vi "Write Running Actors.vi"(6 "Debug Ring Value":u16, 8 "error in (no error)":errorcluster, 10 "Running Actors":refnum<class "CO2 Actor.lvclass">[](array[class]), 11 "cRIO-CO2 in":refnum<class "cRIO-CO2.lvclass">) -> (0 "error out":errorcluster, 3 "cRIO-CO2 out":refnum<class "cRIO-CO2.lvclass">)   [LabVIEW 2015, in "cRIO-Carbondioxide.lvlib" / "cRIO-CO2.lvlib" / "cRIO-CO2.lvclass"]
uses:
  cRIO-CO2.lvclass
  CO2 Actor/CO2 Actor.lvclass
  CO2 Actor/CO2 Actor.lvclass/CO2 Actor.ctl
  <vilib>/ActorFramework/Actor/Actor.lvclass/Actor.ctl
  <vilib>/ActorFramework/Message Enqueuer/Message Enqueuer.lvclass/Message Enqueuer.ctl
  CO2 Actor Messages/Set IndexQ Msg/Set IndexQ Msg.lvclass/Set IndexQ Msg.ctl
  cRIO-CO2.lvclass/cRIO-CO2.ctl
  <vilib>/ActorFramework/Actor/Read Self Enqueuer.vi
  <vilib>/ActorFramework/Message Enqueuer/Enqueue.vi
  <vilib>/ActorFramework/Message Enqueuer/Init from Existing Queue.vi
  <vilib>/ActorFramework/Message Priority Queue/Priority Enqueue.vi
  <vilib>/ActorFramework/Actor/Actor.lvclass
  <vilib>/ActorFramework/Message Enqueuer/Message Enqueuer.lvclass
  CO2 Actor Messages/Set IndexQ Msg/Set IndexQ Msg.lvclass
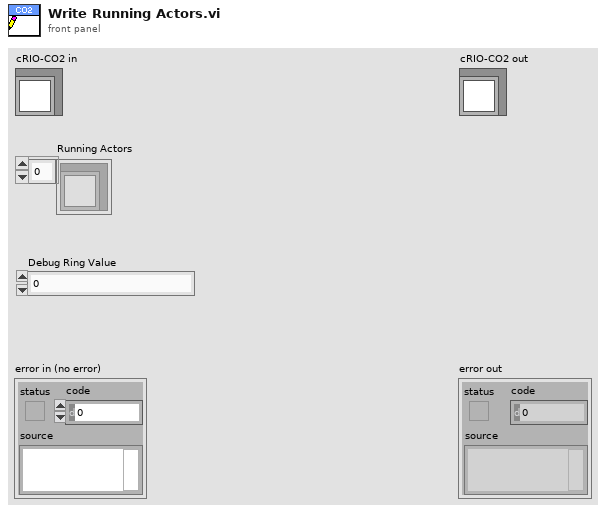
[diagram p1: front panel]
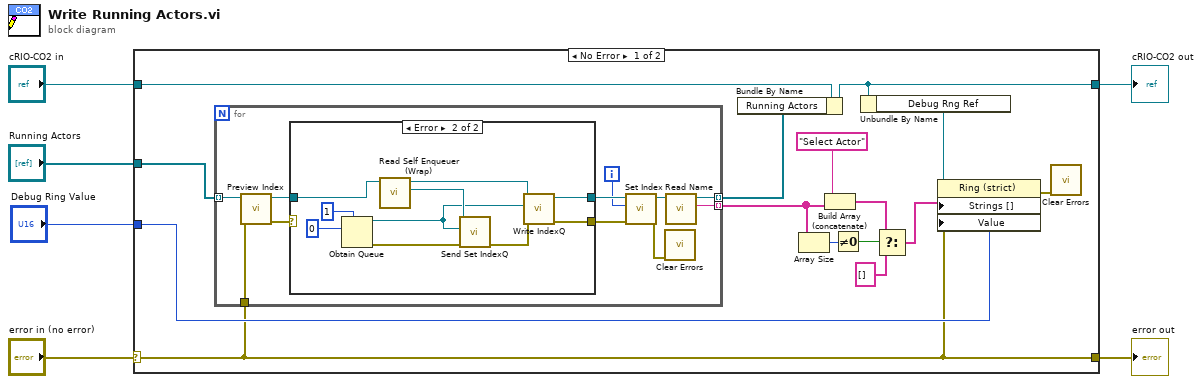
[diagram p0: block diagram]
diagram:
  n1 = case shown="No Error" "error in (no error)" {
    selector: "error in (no error)" -> [w10 w45]
    tunnel: [w10 w45] -> w5
    tunnel: [w8 w46] -> w3
    tunnel: "cRIO-CO2 in" -> [w9 w46]
    tunnel: "Running Actors" -> [w21 _]
    tunnel: "Debug Ring Value" -> [w17 _]
    frame No Error {
      n2 = for {
        tunnel: w21 -> [w29] mode=indexing
        tunnel: [w32] -> w16 mode=indexing
        tunnel: w10 -> [w28]
        tunnel: [w22] -> w7 mode=indexing
        i -> [w23]
        n3 = call "Preview Index.vi"("error in (no error)"=w28, "CO2 Actor in"=w29) -> ("error out"=w27:errorcluster, "CO2 Actor out"=w26:refnum<class "CO2 Actor.lvclass">)  [unwired: 7 in, 1 out]
        n4 = case shown="Error" w27 {
          selector: w27 -> [w33 _]
          tunnel: w26 -> [w34 w42]
          tunnel: [w34 w39] -> w25
          tunnel: [w33 w35] -> w24
          frame No Error {
          }
          frame Error {
            n5 = Obtain Queue(max queue size (-1, unlimited)=1, element data type=0) -> (queue out=w36:refnum<queue>, error out=w37:errorcluster)  [unwired: 3 in, 1 out]
            n6 = call "Read Self Enqueuer (Wrap).vi"("CO2 Actor in"=w42) -> ("Actor Framework:Message Enqueuer"=w41:refnum<class "Message Enqueuer.lvclass">, "CO2 Actor out"=w40:refnum<class "CO2 Actor.lvclass">)  [unwired: 9 in]
            n7 = call "Send Set IndexQ.vi"("error in (no error)"=w37, "IndexQ"=w36, "Message Enqueuer"=w41) -> ("error out"=w38:errorcluster)  [unwired: 7 in, 1 out]
            n8 = call "Write IndexQ.vi"("error in (no error)"=w38, "IndexQ"=w36, "CO2 Actor in"=w40) -> ("error out"=w35:errorcluster, "CO2 Actor out"=w39:refnum<class "CO2 Actor.lvclass">)  [unwired: 7 in]
          }
        }
        n9 = call "Set Index.vi"("error in (no error)"=w24, "Index (-1)"=w23, "CO2 Actor in"=w25) -> ("error out"=w30:errorcluster, "CO2 Actor out"=w31:refnum<class "CO2 Actor.lvclass">)  [unwired: 7 in]
        n10 = call <vilib>:"Clear Errors.vi"("error in (no error)"=w30) -> ()  [unwired: 5 in, 2 out]
        n11 = call "Read Name.vi"("CO2 Actor in"=w31) -> ("Name"=w32:string, "CO2 Actor out"=w22:refnum<class "CO2 Actor.lvclass">)  [unwired: 9 in]
      }
      n12 = Bundle By Name(cluster=w9, "Running Actors"=w7) -> (w8:refnum<class "cRIO-CO2.lvclass">)
      n13 = Array Size(array=w16) -> (size(s)=w15:i32)
      n14 = Build Array (concatenate)("Select Actor", w16) -> (w13:string[])
      n15 = Not Equal To 0?(x=w15) -> (x != 0?=w14:bool)
      n16 = Unbundle By Name(w8) -> ("Debug Rng Ref"=w20:refnum<vi>)
      n17 = Select(t=w13, s=w14, f=string[] []) -> (s? t:f=w12:string[])
      n18 = property class="Ring (strict)"(reference=w20, error in=w10, "Strings []"=w12, "Value"=w17) -> (error out=w19:errorcluster)  [unwired: 1 out]
      n19 = call <vilib>:"Clear Errors.vi"("error in (no error)"=w19) -> ()  [unwired: 5 in, 2 out]
    }
    frame Error {
    }
  }
  "error out" <- w5
  "cRIO-CO2 out" <- w3
